vi "atan2.vi"(10 "Y":dbl[](array[numeric]), 11 "X":dbl[](array[numeric])) -> (3 "atan2":dbl[](array[numeric]))   [LabVIEW 2011]
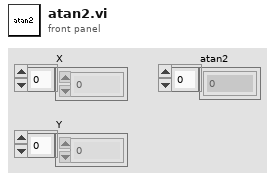
[diagram p1: front panel]
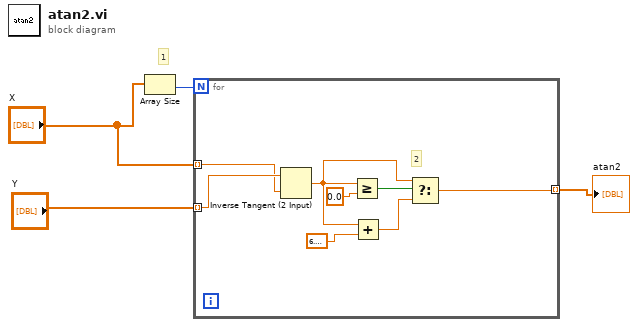
[diagram p0: block diagram]
diagram:
  # "1"
  n1 = Array Size(array="X") -> (size(s)=w3:i32)
  n2 = for {
    N: w3 -> [_]
    tunnel: "Y" -> [w6] mode=indexing
    tunnel: "X" -> [w5] mode=indexing
    tunnel: [w7] -> w1 mode=indexing
    # "2"
    n3 = Inverse Tangent (2 Input)(1:w5, 2:w6) -> (0:w9:dbl)
    n4 = Greater Or Equal?(x=w9, y=0.0) -> (x >= y?=w11:bool)
    n5 = Add(x=w9, y=6.283185307179586) -> (x+y=w10:dbl)
    n6 = Select(t=w9, s=w11, f=w10) -> (s? t:f=w7:dbl)
  }
  "atan2" <- w1
